vi "Get.vi"(11 "String in":refnum<class "String.lvclass">) -> (2 "Value":string)   [LabVIEW 2020, in "Conditum.lvlib" / "Columns.lvlib" / "String.lvclass"]
uses:
  String.lvclass
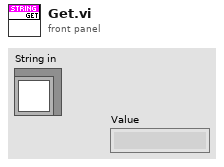
[diagram p1: front panel]
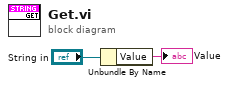
[diagram p0: block diagram]
diagram:
  n1 = Unbundle By Name("String in") -> ("Value"=→"Value":string)
